vi "up_cast.vi"(8 "error in (no error)":errorcluster, 11 "TrajectoryDL091126GenericVoxel in":refnum<class "TrajectoryDL091126GenericVoxel.lvclass">) -> (0 "error out":errorcluster, 3 "GenericTrajectory.lvclass":refnum<class "GenericTrajectory.lvclass">)   [LabVIEW 2010, in "TrajectoryDL091126GenericVoxel.lvclass"]
uses:
  TrajectoryDL091126GenericVoxel.lvclass
  GenericTrajectory/GenericTrajectory/GenericTrajectory.lvclass
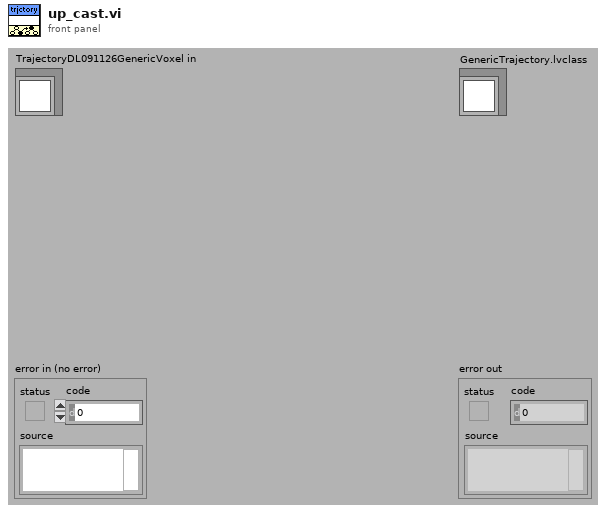
[diagram p1: front panel]
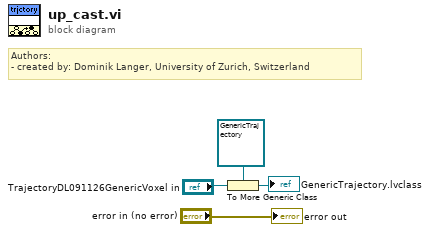
[diagram p0: block diagram]
diagram:
  # "Authors: \n- created by: Dominik Langer, University of Zurich, Switzerland"
  n1 = To More Generic Class(target class=refnum<class "GenericTrajectory.lvclass"> refnum ("GenericTrajectory.lvclass"), reference="TrajectoryDL091126GenericVoxel in") -> (generic class reference=→"GenericTrajectory.lvclass":refnum<class "GenericTrajectory.lvclass">)
  "error out" <- "error in (no error)"
